vi "Init.vi"() -> (3 "Teardown Msg Strategy out":refnum<class "Teardown Msg Strategy.lvclass">)   [LabVIEW 2021, in "jettl.lvlib" / "Teardown Msg Strategy.lvlib" / "Teardown Msg Strategy.lvclass"]
uses:
  Teardown Msg Strategy.lvclass
  Teardown Msg Strategy.lvclass/Teardown Msg Strategy.ctl
  Sender/Sender.lvlib
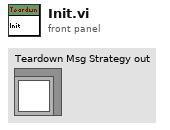
[diagram p1: front panel]
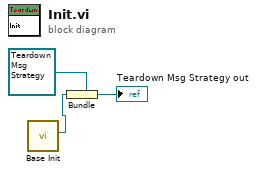
[diagram p0: block diagram]
diagram:
  n1 = call "Base Init.vi"() -> ("Sender"=w1:refnum<class "Sender.lvclass">)  [unwired: 11 in]
  n2 = Bundle "Bundle"(cluster=refnum<class "Teardown Msg Strategy.lvclass"> refnum ("Destroy Msg in"), w1) -> (→"Teardown Msg Strategy out":refnum<class "Teardown Msg Strategy.lvclass">)
